vi "S7COMM - DTL to Timestamp.vi"(8 "error in (no error)":errorcluster, 11 "S7 DTL":u8[](array[numeric]) format="%02x") -> (0 "error out":errorcluster, 1 "Invalid Timestamp":bool, 2 "DTL":T1 {"Weekday" items=["Sunday"=1, "Monday"=2, "Tuesday"=3, "Wednesday"=4, "Thursday"=5, "Friday"=6, "Saturday"=7]; "Month" items=["Jan"=1, "Feb"=2, "Mar"=3, "Apr"=4, "May"=5, "Jun"=6, "Jul"=7, "Aug"=8, "Sep"=9, "Oct"=10, "Nov"=11, "Dec"=12]}, 3 "Time Stamp":timestamp)   [LabVIEW 2014, in "S7NetCom.lvclass"]
uses:
  S7NetCom.lvclass
  S7COMM - DTL--cluster.ctl
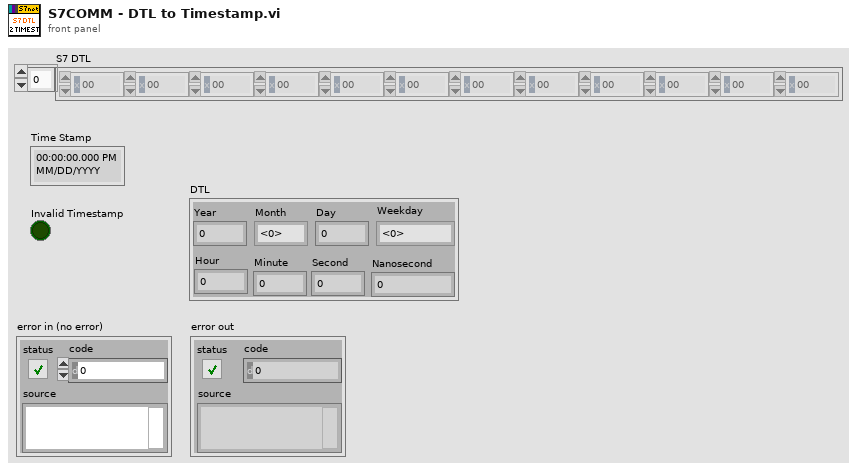
[diagram p1: front panel]
types:
  T1 = typedef "S7NetCom.lvclass/S7COMM - DTL--cluster.ctl" = cluster{"Year":u16, "Month":u8, "Day":u8, "Hour":u8, "Minute":u8, "Second":u8, "Nanosecond":u32, "Weekday":u8}
  T2 = cluster{"fractional second":dbl, "second":i32, "minute":i32, "hour":i32, "day of month":i32, "month":i32, "year":i32, "day of week":i32, "day of year":i32, "DST":i32}
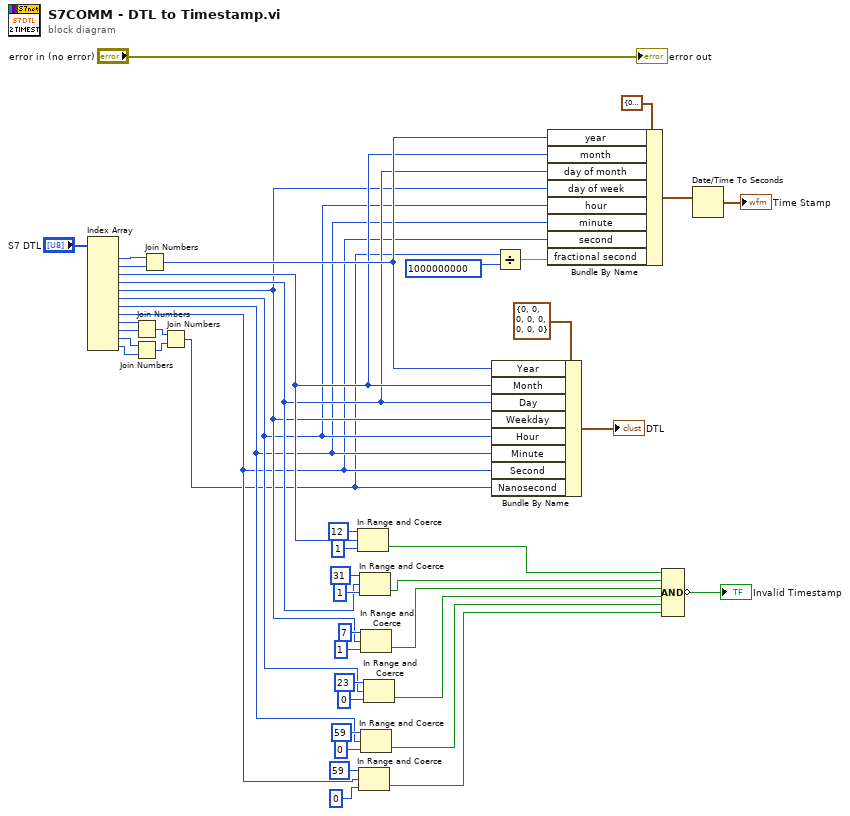
[diagram p0: block diagram]
diagram:
  n1 = Index Array(array="S7 DTL") -> (element #1=w42:u8, element #2=w41:u8, element #3=w10:u8, element #4=w9:u8, element #5=w8:u8, element #6=w7:u8, element #7=w6:u8, element #8=w5:u8, element #9=w26:u8, element #10=w25:u8, element #11=w24:u8, element #12=w23:u8)  [unwired: 12 in]
  n2 = Join Numbers(hi=w26, lo=w25) -> ((hi.lo)=w22:u16)
  n3 = Join Numbers(hi=w24, lo=w23) -> ((hi.lo)=w21:u16)
  n4 = Join Numbers(hi=w42, lo=w41) -> ((hi.lo)=w11:u16)
  n5 = Join Numbers(hi=w22, lo=w21) -> ((hi.lo)=w4:u32)
  n6 = In Range and Coerce(upper limit=u8 12, x=w10, lower limit=u8 1) -> (In Range?=w20:bool)  [unwired: 1 out]
  n7 = In Range and Coerce(upper limit=u8 59, x=w5, lower limit=u8 0) -> (In Range?=w15:bool)  [unwired: 1 out]
  n8 = In Range and Coerce(upper limit=u8 31, x=w9, lower limit=u8 1) -> (In Range?=w19:bool)  [unwired: 1 out]
  n9 = In Range and Coerce(upper limit=u8 7, x=w8, lower limit=u8 1) -> (In Range?=w18:bool)  [unwired: 1 out]
  n10 = In Range and Coerce(upper limit=u8 59, x=w6, lower limit=u8 0) -> (In Range?=w16:bool)  [unwired: 1 out]
  n11 = In Range and Coerce(upper limit=u8 23, x=w7, lower limit=u8 0) -> (In Range?=w17:bool)  [unwired: 1 out]
  n12 = Bundle By Name(cluster=T1 {"Year"=0, "Month"=0, "Day"=0, "Hour"=0, "Minute"=0, "Second"=0, "Nanosecond"=0, "Weekday"=0} ("S7 Date & Time"), "Year"=w11, "Month"=w10, "Day"=w9, "Weekday"=w8, "Hour"=w7, "Minute"=w6, "Second"=w5, "Nanosecond"=w4) -> (→"DTL":T1)
  n13 = Divide(x=w4, y=u32 1000000000) -> (x/y=w2:dbl)
  n14 = Bundle By Name(cluster=T2 {"fractional second"=0.0, "second"=0, "minute"=0, "hour"=0, "day of month"=0, "month"=0, "year"=0, "day of week"=0, "day of year"=0, "DST"=0} ("date time rec"), "year"=w11, "month"=w10, "day of month"=w9, "day of week"=w8, "hour"=w7, "minute"=w6, "second"=w5, "fractional second"=w2) -> (w13:T2)
  n15 = Compound Arithmetic op=AND(w20, w19, w18, w17, w16, w15) -> (invert →"Invalid Timestamp":bool)
  n16 = Date/Time To Seconds(2:w13) -> (0:→"Time Stamp":timestamp)  [unwired: 1 in]
  "error out" <- "error in (no error)"
